vi "BRig_dataAnalog_iState_end.vi"() -> (2 "output_iState_end":i32)   [LabVIEW 2014]
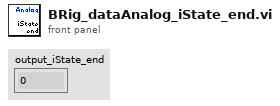
[diagram p1: front panel]
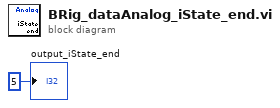
[diagram p0: block diagram]
diagram:
  "output_iState_end" <- 5 ("output_iBlock")
